vi "Check_Enable_Cycling_Flag.vi"(8 "error in (no error)":errorcluster, 11 "Data Cluster in":T1 {"VestaTemperature"."Water Heater Temp (°F)" min=32 max=203}) -> (0 "error out":errorcluster, 3 "Data Cluster out":T1 {"VestaTemperature"."Water Heater Temp (°F)" min=32 max=203}, 4 "Send_Vesta_Message":u8, 6 "Send_Timer_Message":u8)   [LabVIEW 2023]
uses:
  Drivers/Resideo Gas Valve/Type Definitions/Vesta Info.ctl
  Drivers/Resideo Gas Valve/Type Definitions/Temperature Control.ctl
  controls/Burner Duty Cycle.ctl
  controls/Timer Application Cluster.ctl
  controls/UI Data.ctl
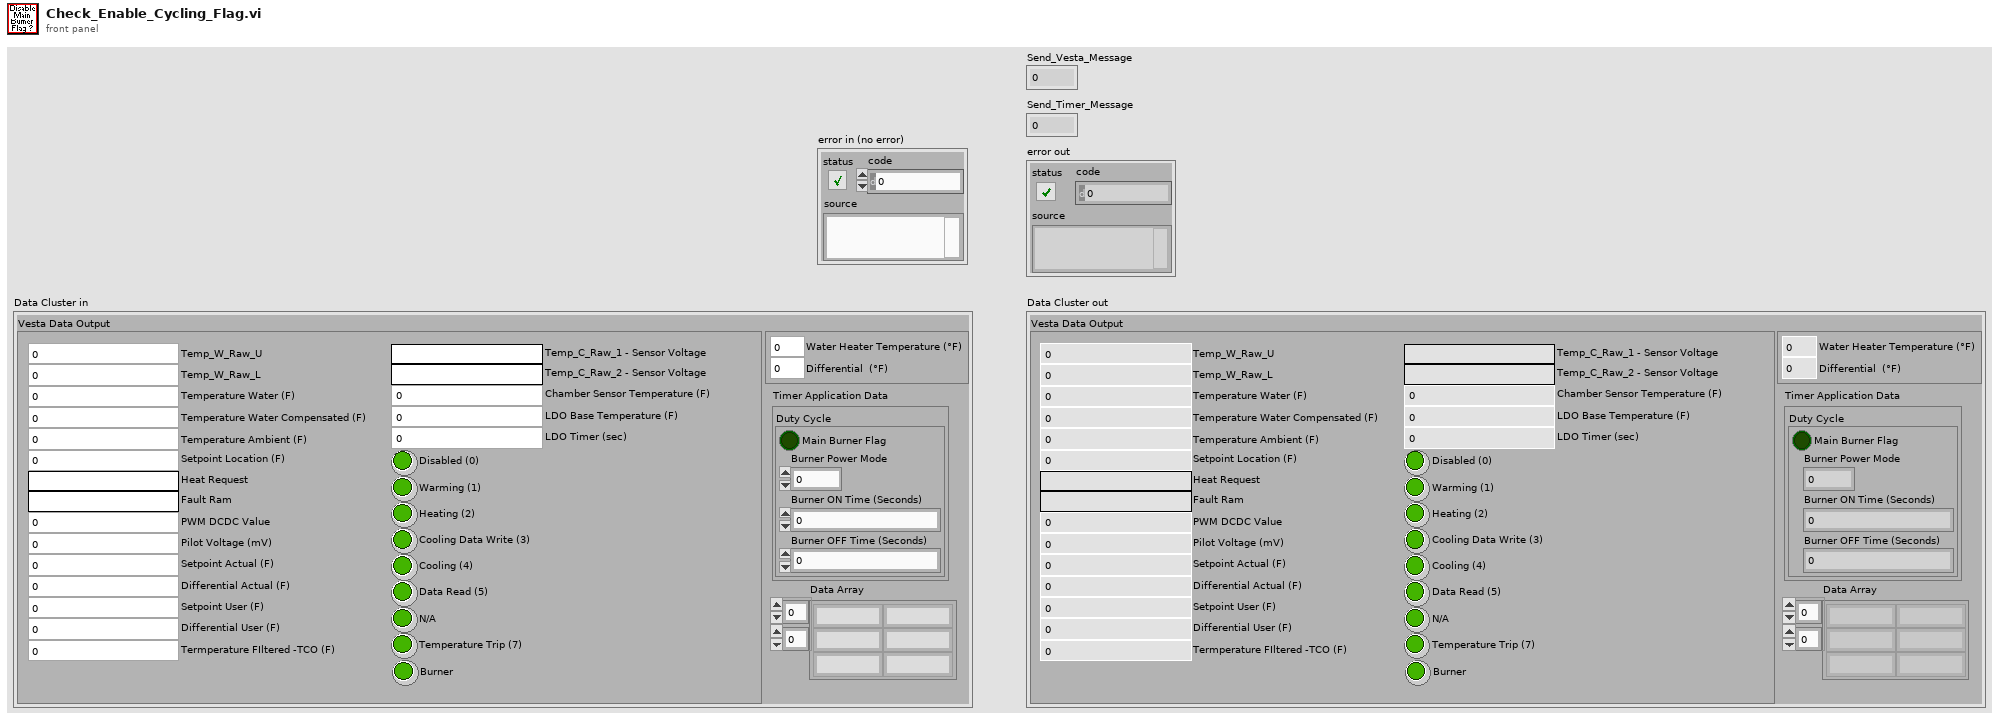
[diagram p1: front panel]
types:
  T1 = typedef "UI Data.ctl" = cluster{"Vesta Data Output":T2, "VestaTemperature":T3, "Timer Application Data":T4, "Data Array":string[][]}
  T2 = typedef "Vesta Info.ctl" = cluster{"Temp_W_Raw_U":u16, "Temp_W_Raw_L":u16, "Temperature Water (F)":dbl, "Temperature Water Compensated (F)":dbl, "Temperature Ambient (F)":dbl, "Setpoint Location (F)":dbl, "Heat Request":string, "Fault Ram":string, "PWM DCDC Value":u16, "Pilot Voltage (mV)":dbl, "Setpoint Actual (F)":dbl, "Differential Actual (F)":dbl, "Setpoint User (F)":dbl, "Differential User (F)":dbl, "Termperature FIltered -TCO (F)":dbl, "Temp_C_Raw_1 - Sensor Voltage":string, "Temp_C_Raw_2 - Sensor Voltage":string, "Chamber Sensor Temperature (F)":dbl, "LDO Base Temperature (F)":dbl, "LDO Timer (sec)":i16, "Disabled (0)":bool, "Warming (1)":bool, "Heating (2)":bool, "Cooling Data Write (3)":bool, "Cooling (4)":bool, "Data Read (5)":bool, "N/A":bool, "Temperature Trip (7)":bool, "Burner":bool}
  T3 = typedef "Temperature Control.ctl" = cluster{"Water Heater Temp (°F)":u16, "Differential  (°F)":dbl}
  T4 = typedef "Timer Application Cluster.ctl" = cluster{"Duty Cycle":T5}
  T5 = typedef "Burner Duty Cycle.ctl" = cluster{"Burner ON Time (Seconds)":dbl, "Burner OFF Time (Seconds)":dbl, "Main Burner Flag":bool, "Burner Power Mode":u8}
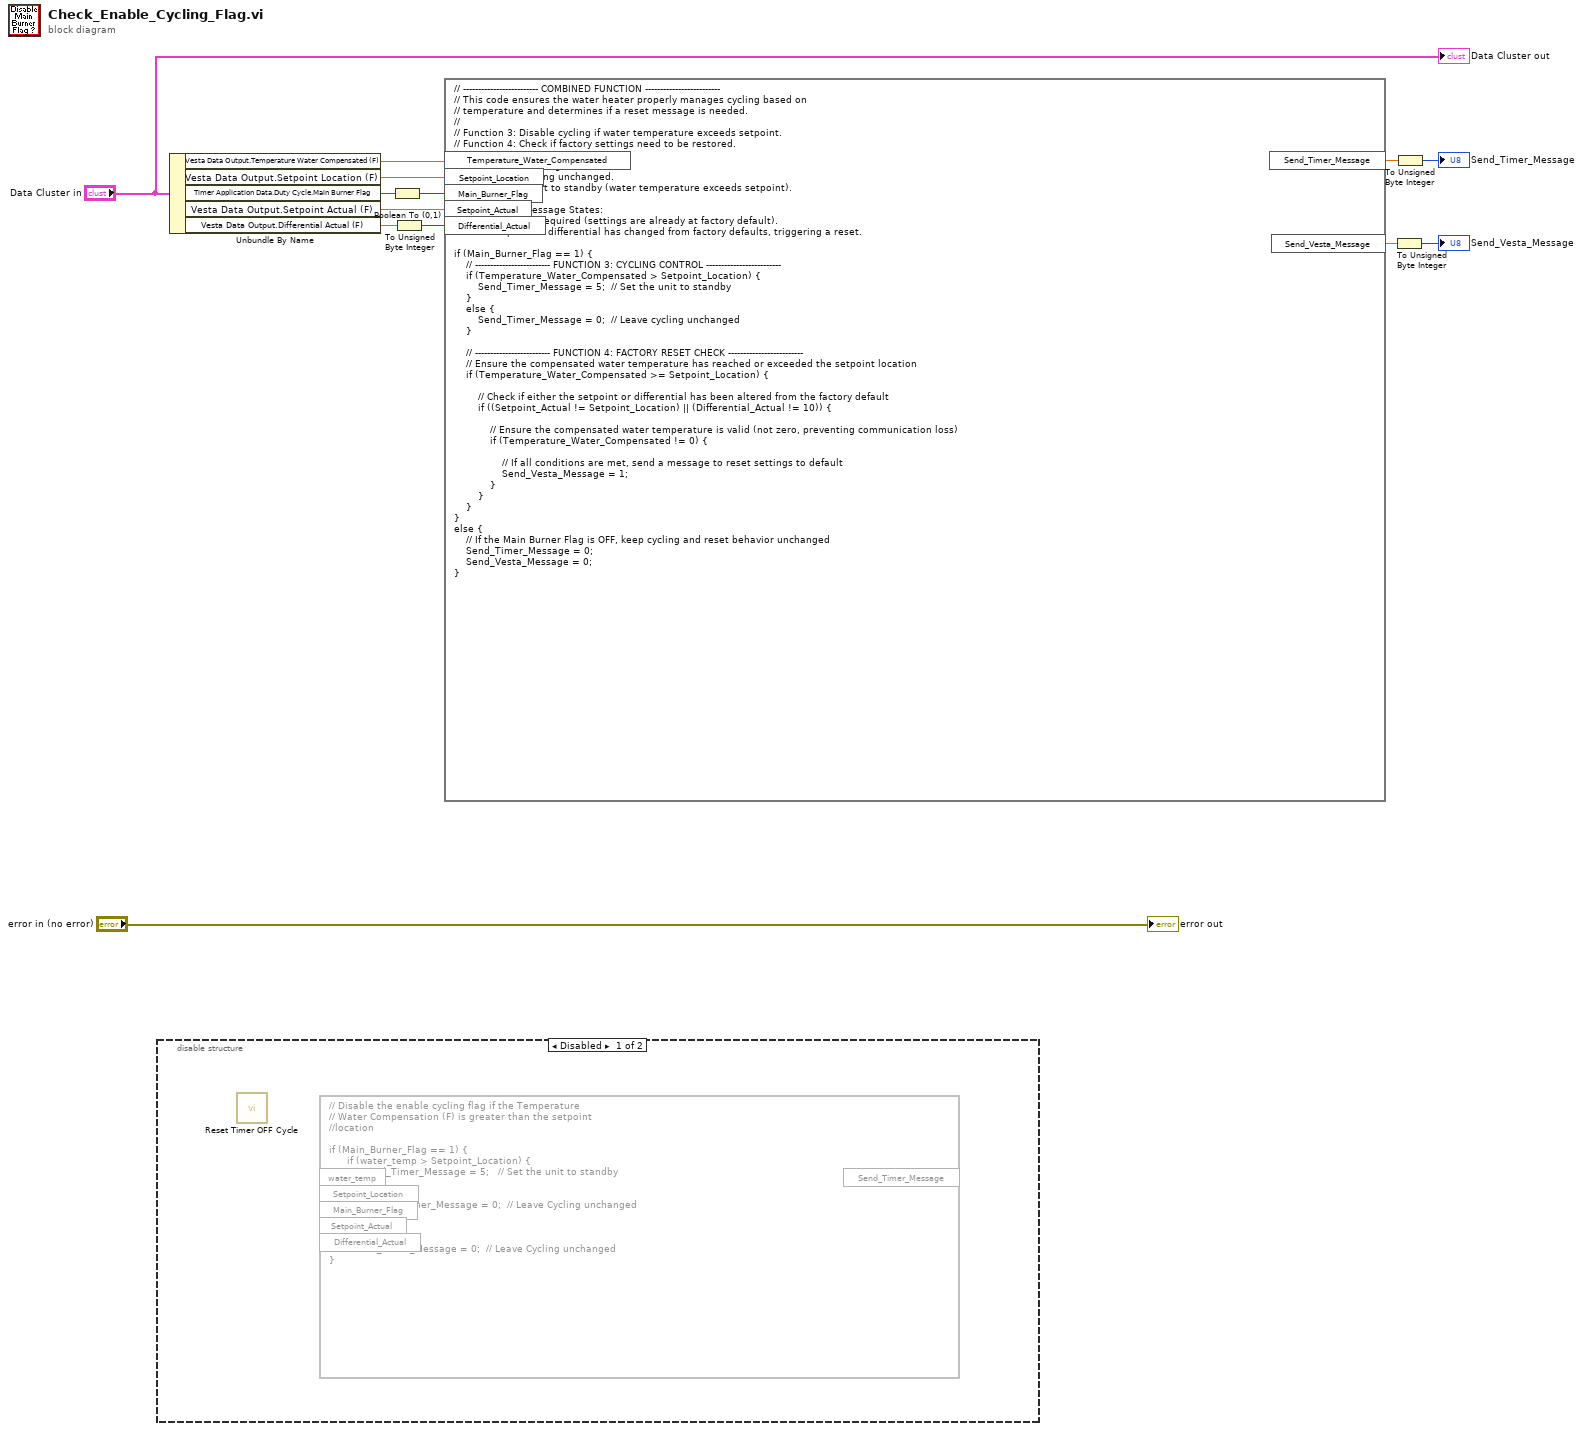
[diagram p0: block diagram]
diagram:
  n1 = disable-structure shown="Disabled" {
    frame Disabled {
      n2 = call "Reset Timer OFF Cycle.vi"() -> ()  [unwired: 11 in, 1 out]
      n3 = formula code="// Disable the enable cycling flag if the Temperature\n// Water Compensation (F) is greater than the setpoint\n//location\n\nif (Main_Burner_Flag == 1) {\n      if (water_temp > Setpoint_Location) {\n           Send_Timer_Message = 5;   // Set the unit to standby\n         }\n      else {\n               Send_Timer_Message = 0;  // Leave Cycling unchanged\n              }  \n   }\nelse {\n        Send_Timer_Message = 0;  // Leave Cycling unchanged\n}"() -> ()  [unwired: 5 in, 1 out]
    }
    frame Enabled {
    }
  }
  n4 = Unbundle By Name("Data Cluster in") -> ("Vesta Data Output.Temperature Water Compensated (F)"=w12:dbl, "Vesta Data Output.Setpoint Location (F)"=w13:dbl, "Timer Application Data.Duty Cycle.Main Burner Flag"=w11:bool, "Vesta Data Output.Setpoint Actual (F)"=w5:dbl, "Vesta Data Output.Differential Actual (F)"=w4:dbl)
  n5 = Boolean To (0,1)(Boolean=w11) -> (0, 1=w9:i16)
  n6 = To Unsigned Byte Integer(number=w4) -> (unsigned 8bit integer=w3:u8)
  n7 = formula code="// ------------------------- COMBINED FUNCTION -------------------------\n// This code ensures the water heater properly manages cycling based on  \n// temperature and determines if a reset message is needed.  \n//\n// Function 3: Disable cycling if water temperature exceeds setpoint.  \n// Function 4: Check if factory settings need to be restored.\n//\n// Send_Timer_Message States:\n// - `0`: Leave cycling unchanged.  \n// - `5`: Set the unit to standby (water temperature exceeds setpoint).  \n//\n// Send_Vesta_Message States:\n// - `0`: No action required (settings are already at factory default).  \n// - `1`: Setpoint or differential has changed from factory defaults, triggering a reset.  \n\nif (Main_Burner_Flag == 1) {\n    // ------------------------- FUNCTION 3: CYCLING CONTROL -------------------------\n    if (Temperature_Water_Compensated > Setpoint_Location) {\n        Send_Timer_Message = 5;  // Set the unit to standby\n    } \n    else {\n        Send_Timer_Message = 0;  // Leave cycling unchanged\n    }\n\n    // ------------------------- FUNCTION 4: FACTORY RESET CHECK -------------------------\n    // Ensure the compensated water temperature has reached or exceeded the setpoint location\n    if (Temperature_Water_Compensated >= Setpoint_Location) {  \n        \n        // Check if either the setpoint or differential has been altered from the factory default\n        if ((Setpoint_Actual != Setpoint_Location) || (Differential_Actual != 10)) {  \n\n            // Ensure the compensated water temperature is valid (not zero, preventing communication loss)\n            if (Temperature_Water_Compensated != 0) {  \n                \n                // If all conditions are met, send a message to reset settings to default\n                Send_Vesta_Message = 1;  \n            }\n        }\n    }\n} \nelse {\n    // If the Main Burner Flag is OFF, keep cycling and reset behavior unchanged\n    Send_Timer_Message = 0;\n    Send_Vesta_Message = 0;\n}"("Temperature_Water_Compensated"=w12, "Setpoint_Location"=w13, "Main_Burner_Flag"=w9, "Setpoint_Actual"=w5, "Differential_Actual"=w3) -> ("Send_Timer_Message"=w10:dbl, "Send_Vesta_Message"=w1:dbl)
  n8 = To Unsigned Byte Integer(number=w1) -> (unsigned 8bit integer=→"Send_Vesta_Message":u8)
  n9 = To Unsigned Byte Integer(number=w10) -> (unsigned 8bit integer=→"Send_Timer_Message":u8)
  "error out" <- "error in (no error)"
  "Data Cluster out" <- "Data Cluster in"
